vi "ECOG-Build.vi"() -> ()   [LabVIEW 2020]
uses:
  Typedefs/ECOG-Globals.vi
panel:
  out "Version":string="0.1-alpha.0"
  out "Progress Bar":u8(slide) caption="Error" scale=0.0..5.0
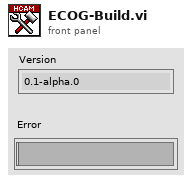
[diagram p1: front panel]
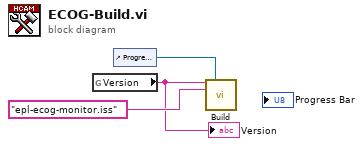
[diagram p0: block diagram]
diagram:
  n1 = global read "ECOG-Globals.vi" "Version"() -> (w1:string)
  "Version" <- w1
  n2 = control-ref of="Progress Bar"() -> (w2:refnum<vi>)
  n3 = call "Build.vi"("version"=w1, "Progress Bar"=w2, "iss path"="epl-ecog-monitor.iss") -> ()  [unwired: 13 in]
